vi "Angular PID Controller.vi"(8 "error in":errorcluster) -> ()   [LabVIEW 2015]
doc: "This VI executes continuously carrying out the current operation and responding to updates or new operations. It will often contain the timing or control code that is difficult to place directly in TeleOp. This VI generally opens all sensors and motors and isolates the rest of the robot code from knowing how the operations are carried out."
uses:
  <vilib>/Rock Robotics/WPI/CAN/TalonSRX/WPI_CANTalonSRX_GlobalStatus.ctl
  <vilib>/Rock Robotics/WPI/MotorControl/WPI_MotorControlOpenCANTalonSRX.vi
  Angular PID Setpoints.ctl
  Angular PID Operations.ctl
  <vilib>/Rock Robotics/WPI/CAN/TalonSRX/WPI_CANTalonSRX_APIControlMode.ctl
  <vilib>/Rock Robotics/WPI/CAN/TalonSRX/WPI_CANTalonSRX_APIFeedbackSelect.ctl
  <vilib>/Rock Robotics/Network Tables/NT Write Boolean.vi
panel:
  out "Out F":dbl
  out "Out I Zone":dbl
  out "Out Ramp Rate":dbl
  out "Out D":dbl
  out "Out I":dbl
  out "Out P":dbl
  in  "Ramp Rate":dbl format="%#_13g"
  in  "I Zone":dbl format="%#_13g"
  in  "F":dbl format="%#_13g"
  in  "D":dbl format="%#_13g"
  in  "I":dbl=0.03 format="%#_13g"
  in  "P":dbl=3.0 format="%#_13g"
  in  "Update PID":bool
  out "Talon SRX Status 2":T1
  out "Current Rev":dbl
  out "Talon SRX Status":T1
  out "Set OutPut":dbl
  out "Current\nCmd":string
  # "Tip: It may be helpful to observe inputs and sensor values.\nYou may also want to display tuning or debugging controls."
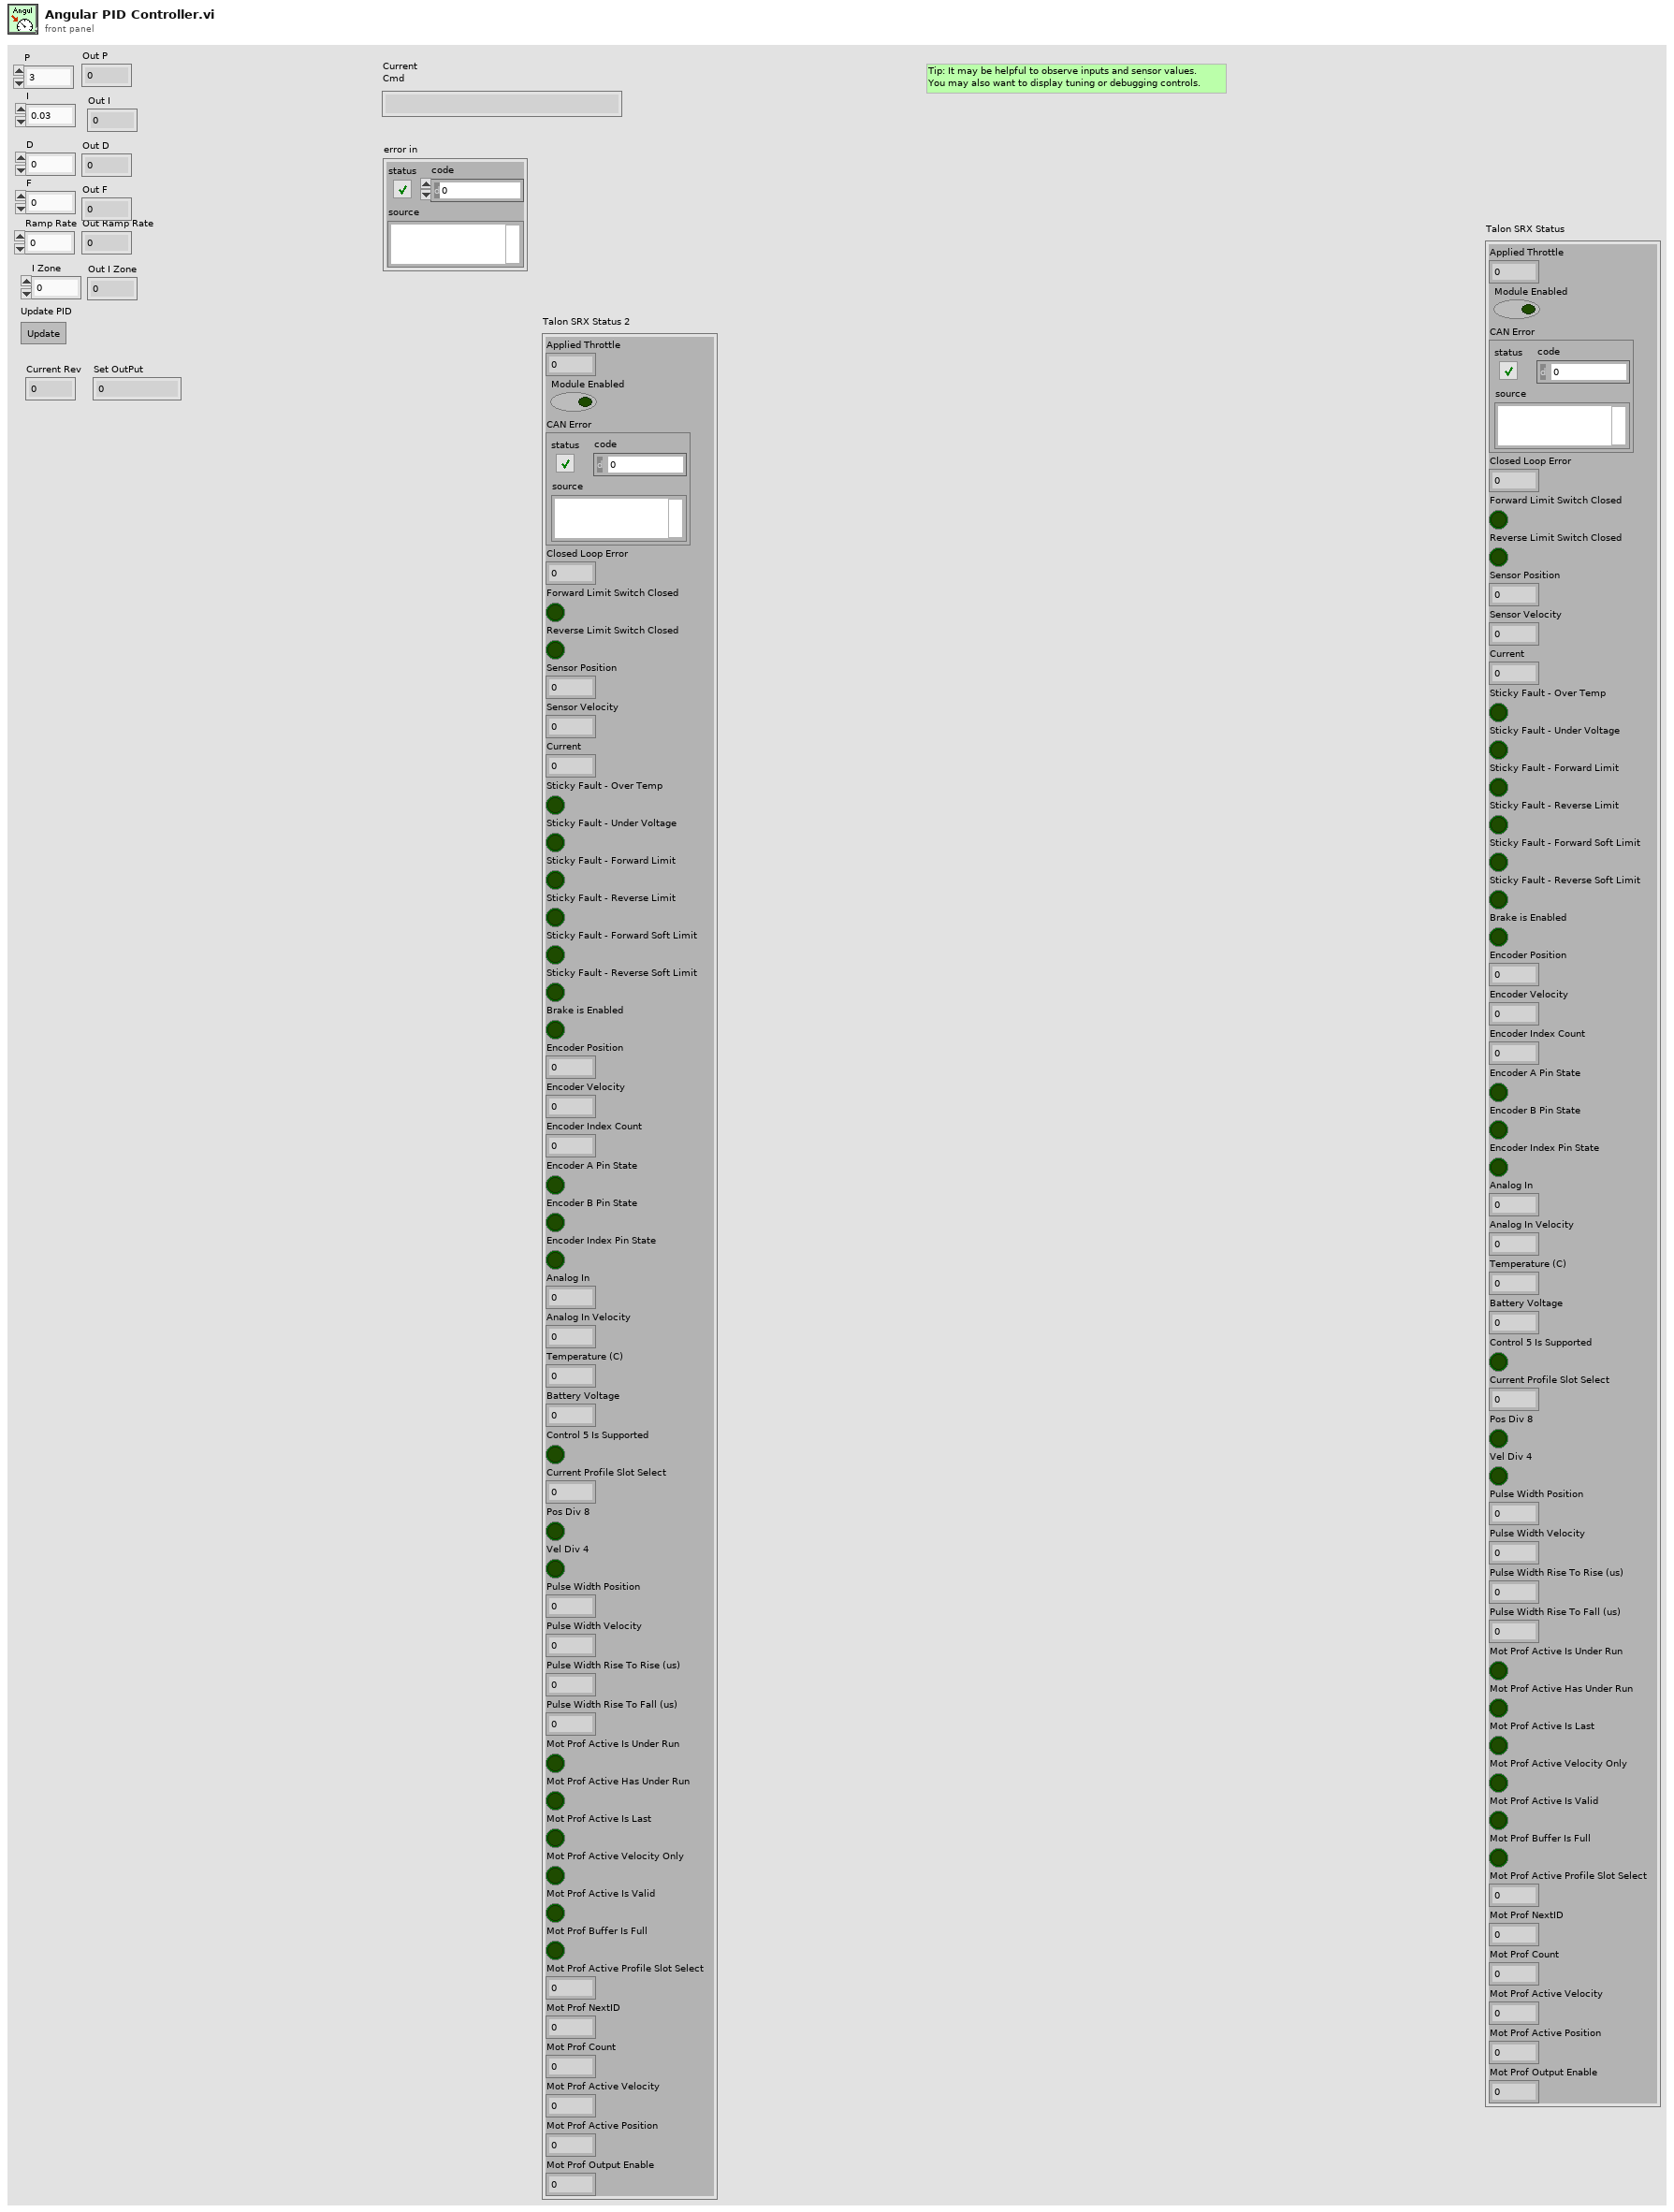
[diagram p1: front panel]
types:
  T1 = typedef "WPI_CANTalonSRX_GlobalStatus.ctl" = cluster{"Applied Throttle":dbl, "Module Enabled":bool, "CAN Error":errorcluster, "Closed Loop Error":dbl, "Forward Limit Switch Closed":bool, "Reverse Limit Switch Closed":bool, "Sensor Position":dbl, "Sensor Velocity":dbl, "Current":dbl, "Sticky Fault - Over Temp":bool, "Sticky Fault - Under Voltage":bool, "Sticky Fault - Forward Limit":bool, "Sticky Fault - Reverse Limit":bool, "Sticky Fault - Forward Soft Limit":bool, "Sticky Fault - Reverse Soft Limit":bool, "Brake is Enabled":bool, "Encoder Position":dbl, "Encoder Velocity":dbl, "Encoder Index Count":dbl, "Encoder A Pin State":bool, "Encoder B Pin State":bool, "Encoder Index Pin State":bool, "Analog In":dbl, "Analog In Velocity":dbl, "Temperature (C)":dbl, "Battery Voltage":dbl, "Control 5 Is Supported":bool, "Current Profile Slot Select":dbl, "Pos Div 8":bool, "Vel Div 4":bool, "Pulse Width Position":i32, "Pulse Width Velocity":i32, "Pulse Width Rise To Rise (us)":i32, "Pulse Width Rise To Fall (us)":i32, "Mot Prof Active Is Under Run":bool, "Mot Prof Active Has Under Run":bool, "Mot Prof Active Is Last":bool, "Mot Prof Active Velocity Only":bool, "Mot Prof Active Is Valid":bool, "Mot Prof Buffer Is Full":bool, "Mot Prof Active Profile Slot Select":i32, "Mot Prof NextID":i32, "Mot Prof Count":i32, "Mot Prof Active Velocity":dbl, "Mot Prof Active Position":dbl, "Mot Prof Output Enable":i32}
  T2 = typedef "WPI_CANTalonSRX_APIFeedbackSelect.ctl" = enum16{"Digital Quadrature Encoder", "Analog Potentiometer", "Analog Encoder", "Count on Quad-A (Rising-Edge)", "Count on Quad-A (Falling-Edge)", "CTR Magnetic Enc (Absolute)", "CTR Magnetic Enc (Relative)", "Pulse Width"}
  T3 = typedef "WPI_CANTalonSRX_APIControlMode.ctl" = enum8{"Percent VBus", "Speed", "Position", "Slave", "Unchanged / Invalid", "Voltage Compensation", "Current", "Motion Profile"}
  T4 = typedef "Angular PID Setpoints.ctl" = cluster{"Operation":T5, "Setpoint":dbl, "Duration":dbl}
  T5 = typedef "Angular PID Operations.ctl" = enum16{"Reserve", "Read Current", "Immediate", "Turn To Angle"}
  T6 = typedef "WPI_MotorControlDeviceRef.ctl" = cluster{"DeviceStatus":errorcluster, "Type":T7, "PWM":cluster{"PWM Channel":T8, "DeadBand":T9}, "CAN":cluster{"Device Number":u8, "Control Mode":T10, "Semaphore":T11, "Max Vout":dbl, "TalonSRX Control Mode":T3}, "Invert":bool}
  T7 = typedef "WPI_MotorControlType.ctl" = enum16{"PWM", "CAN", "CANTalonSRX"}
  T8 = typedef "FPGA_DIOPWMChannel.ctl" = enum8{"PWM 0", "PWM 1", "PWM 2", "PWM 3", "PWM 4", "PWM 5", "PWM 6", "PWM 7", "PWM 8", "PWM 9", "PWM MXP 0", "PWM MXP 1", "PWM MXP 2", "PWM MXP 3", "PWM MXP 4", "PWM MXP 5", "PWM MXP 6", "PWM MXP 7", "PWM MXP 8", "PWM MXP 9", "Invalid"}
  T9 = typedef "WPI_PWMDeadband.ctl" = cluster{"Name":string, "maxPositivePwm":i32, "minPositivePwm":i32, "centerPwm":i32, "maxNegativePwm":i32, "minNegativePwm":i32, "angularRange":u16}
  T10 = typedef "WPI_CANJaguar_ControlMode.ctl" = enum8{"Percent VBus", "Current", "Speed", "Position", "Voltage"}
  T11 = typedef "Semaphore RefNum" = refnum<k1>
  T12 = typedef "Command Status Info.ctl" = cluster{"Name":string, "Status":T13, "notifier out":T14}
  T13 = typedef "Completion Status.ctl" = enum16{"Successful", "Aborted", "Incomplete"}
  T14 = typedef "Completion Notifier.ctl" = refnum<notifier>
  T15 = cluster{"Default Command":T4, "Command Timing":cluster{"Start Time (ms)":u32, "Iterations":i32}, "Command Arguments":cluster{"Command Info":T12, "Description":string, "Default Command":T4, "notifier out":refnum<notifier>, "Subsystem Name":string}}
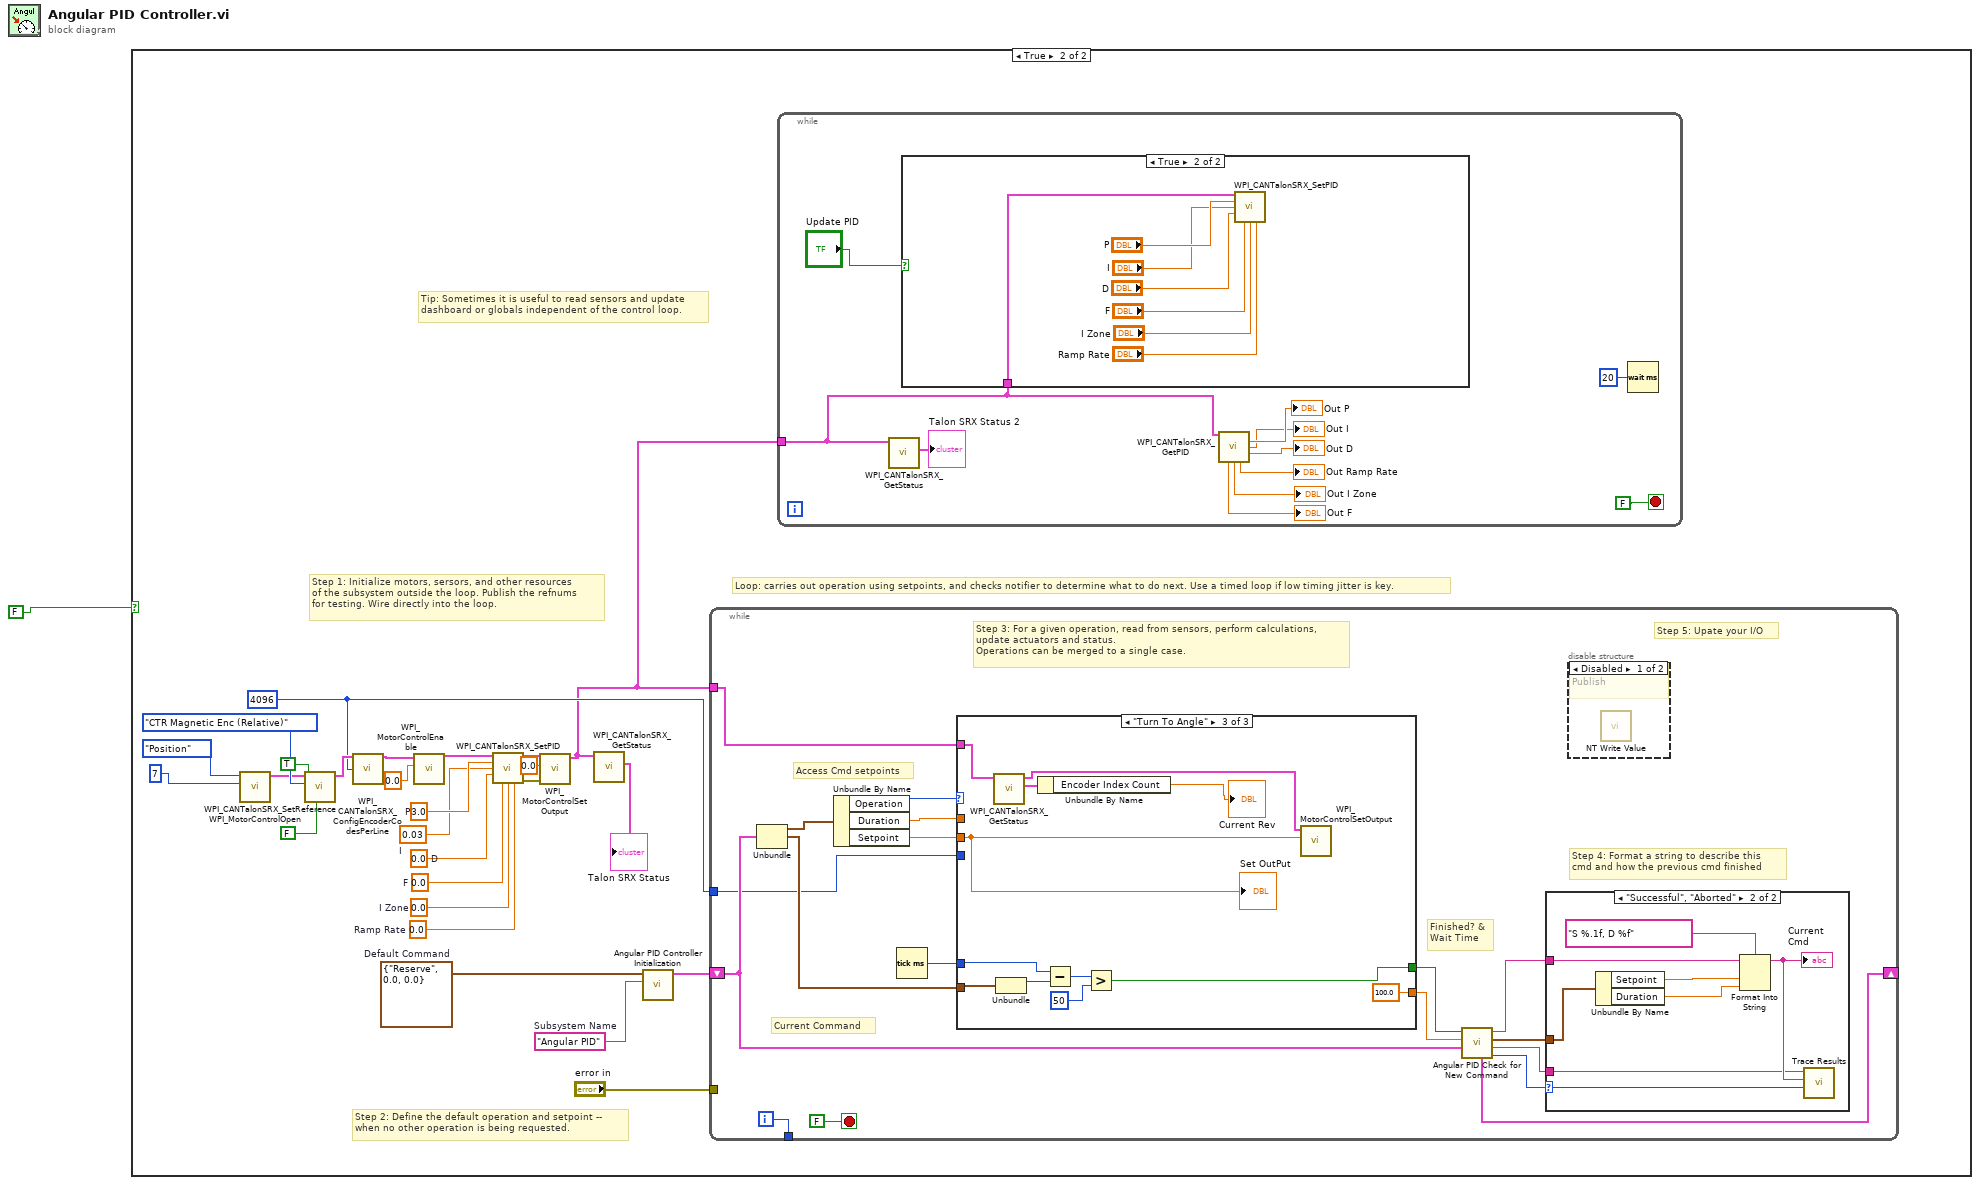
[diagram p0: block diagram]
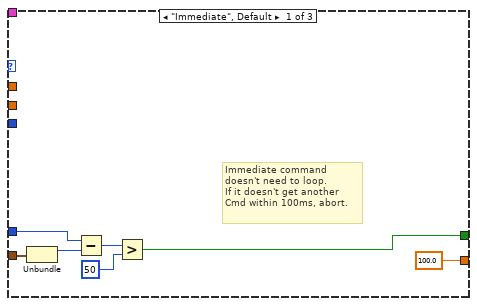
[diagram p6: hidden frame]
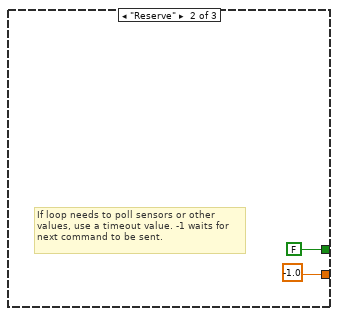
[diagram p7: hidden frame]
diagram:
  n1 = case shown="True" FALSE {
    frame False {
    }
    frame True {
      w10 = 0.0  # Ramp Rate
      w11 = 0.0  # I Zone
      w12 = 0.0  # F
      w13 = 0.0  # D
      w14 = 0.03  # I
      w15 = 3.0  # P
      w8 = u32 4096 ("Number Encoder Lines\n(Counts Per Rotation)")
      w24 = T4 {"Operation"=enum."Reserve", "Setpoint"=0.0, "Duration"=0.0}  # Default Command
      w25 = "Angular PID"  # Subsystem Name
      # "Tip: Sometimes it is useful to read sensors and update\ndashboard or globals independent of the control loop."
      # "Step 2: Define the default operation and setpoint --\nwhen no other operation is being requested."
      # "Step 1: Initialize motors, sersors, and other resources\nof the subsystem outside the loop. Publish the refnums\nfor testing. Wire directly into the loop."
      # "Loop: carries out operation using setpoints, and checks notifier to determine what to do next. Use a timed loop if low timing jitter is key."
      n2 = call-poly <vilib>:"WPI_MotorControlOpen.vi"("Device Number"=u8 7, "Control Mode"=WPI_CANTalonSRX_APIControlMode."Position") -> ("MotorControlDeviceRef"=w20:T6)  [unwired: 8 in, 1 out]
      n3 = call <vilib>:"WPI_CANTalonSRX_SetReference.vi"("Reverse Closed-Loop Output"=FALSE, "Reverse Feedback Sensor"=TRUE, "Feedback Reference"=WPI_CANTalonSRX_APIFeedbackSelect."CTR Magnetic Enc (Relative)", "CAN Talon SRX Ref"=w20) -> ("CAN Talon SRX Ref"=w19:T6)  [unwired: 6 in, 1 out]
      n4 = call <vilib>:"WPI_CANTalonSRX_ConfigEncoderCodesPerLine.vi"("CAN Talon SRX Ref"=w19, "Number Encoder Lines\n(Counts Per Rotation)"=w8) -> ("CAN Talon SRX Ref"=w18:T6)  [unwired: 12 in, 1 out]
      n5 = call <vilib>:"WPI_MotorControlEnable.vi"("Encoder Initial Position"=0.0, "CAN MotorDevRef"=w18) -> ("CAN MotorDevRef"=w16:T6)  [unwired: 8 in, 1 out]
      n6 = call <vilib>:"WPI_CANTalonSRX_SetPID.vi"("CAN Talon SRX Ref"=w16, "P"=w15, "I"=w14, "D"=w13, "F"=w12, "I Zone"=w11, "Ramp Rate"=w10) -> ("CAN Talon SRX Ref"=w6:T6, "error out"=w7:errorcluster)  [unwired: 7 in]
      n7 = call <vilib>:"WPI_MotorControlSetOutput.vi"("error in (no error)"=w7, "Output"=0.0, "MotorControlDevRef"=w6) -> ("MotorControlDevRef"=w3:T6)  [unwired: 6 in, 2 out]
      n8 = call <vilib>:"WPI_CANTalonSRX_GetStatus.vi"("CAN Talon SRX Ref"=w3) -> ("Talon SRX Status"=→"Talon SRX Status":T1)  [unwired: 8 in, 2 out]
      n9 = call "Angular PID Controller Initialization.vi"("Subsystem Name"=w25, "Default Command"=w24) -> ("Command Info"=w26:T15)  [unwired: 9 in]
      n10 = while {
        shift-right: [w54] -> _
        shift-left: w26 -> [w55]
        tunnel: [w62] -> _
        tunnel: "error in" -> [_]
        tunnel: w3 -> [w47]
        tunnel: w8 -> [w46]
        i -> [w62]
        stop <- FALSE stop-if-true
        # "Step 5: Upate your I/O"
        # "Step 4: Format a string to describe this\ncmd and how the previous cmd finished"
        # "Current Command"
        # "Access Cmd setpoints"
        # "Finished? &\nWait Time"
        # "Step 3: For a given operation, read from sensors, perform calculations,\nupdate actuators and status.\nOperations can be merged to a single case."
        n11 = Unbundle(w55) -> ("Default Command"=w61:T4, "Command Timing"=w57:cluster{"Start Time (ms)":u32, "Iterations":i32})  [unwired: 1 out]
        n12 = Unbundle By Name(w61) -> ("Operation"=w60:T5, "Duration"=w59:dbl, "Setpoint"=w56:dbl)
        n13 = Tick Count (ms)() -> (millisecond timer value=w58:u32)
        n14 = case shown="\"Turn To Angle\"" w60 {
          tunnel: [100.0 -1.0 100.0] -> w52
          tunnel: [w72 FALSE ("ignore previous (F)") w81] -> w53
          tunnel: w57 -> [w74 _ w82]
          tunnel: w59 -> [_ _ _]
          tunnel: w58 -> [w73 _ w83]
          tunnel: w56 -> [_ _ w89]
          tunnel: w47 -> [_ _ w91]
          tunnel: w46 -> [_ _ _]
          frame "Immediate", Default {
            # "Immediate command\ndoesn't need to loop.\nIf it doesn't get another\nCmd within 100ms, abort."
            n15 = Unbundle(w74) -> ("Start Time (ms)"=w77:u32)  [unwired: 1 out]
            n16 = Subtract(x=w73, y=w77) -> (x-y=w76:u32)
            n17 = Greater?(x=w76, y=u8 50 ("Left Motor")) -> (0:w72:bool)
          }
          frame "Reserve" {
            # "If loop needs to poll sensors or other\nvalues, use a timeout value. -1 waits for\nnext command to be sent."
          }
          frame "Turn To Angle" {
            n18 = call <vilib>:"WPI_CANTalonSRX_GetStatus.vi"("CAN Talon SRX Ref"=w91) -> ("Talon SRX Status"=w90:T1, "CAN Talon SRX Ref"=w88:T6)  [unwired: 8 in, 1 out]
            n19 = Unbundle(w82) -> ("Start Time (ms)"=w86:u32)  [unwired: 1 out]
            n20 = Unbundle By Name(w90) -> ("Encoder Index Count"=→"Current Rev":dbl)
            n21 = Subtract(x=w83, y=w86) -> (x-y=w85:u32)
            n22 = Greater?(x=w85, y=u8 50 ("Left Motor")) -> (0:w81:bool)
            n23 = call <vilib>:"WPI_MotorControlSetOutput.vi"("Output"=w89, "MotorControlDevRef"=w88) -> ()  [unwired: 7 in, 3 out]
            "Set OutPut" <- w89
          }
        }
        n24 = call "Angular PID Check for New Command.vi"("Current Command"=w55, "Wait time (ms)"=w52, "Finished?"=w53) -> ("Completion"=w48:T13, "Subsystem Name"=w49:string, "Current Command"=w50:T4, "Initial Trace String"=w51:string, "NextCommand"=w54:T15)  [unwired: 4 in]
        n25 = case shown="\"Successful\", \"Aborted\"" w48 {
          selector: w48 -> [_ w71]
          tunnel: w51 -> [_ w67]
          tunnel: w50 -> [_ w68]
          tunnel: w49 -> [_ w64]
          frame "Incomplete", Default {
            # "Continuing current command"
          }
          frame "Successful", "Aborted" {
            # "Report and setup for next command"
            n26 = Unbundle By Name(w68) -> ("Setpoint"=w70:dbl, "Duration"=w65:dbl)
            n27 = Format Into String(format string="S %.1f, D %f", initial string=w67, w70, w65) -> (resulting string=w66:string)  [unwired: 1 in, 1 out]
            "Current\nCmd" <- w66
            n28 = call <vilib>:"Trace Results.vi"("Status of previous command"=w71, "Description"=w66, "Subsystem"=w64) -> ()  [unwired: 9 in]
          }
        }
        n29 = disable-structure shown="Disabled" {
          frame Disabled {
            # "Publish"
            n30 = call-poly <vilib>:"NT Write Value.vi"() -> ()  [unwired: 11 in, 1 out]
          }
          frame Enabled {
          }
        }
      }
      n31 = while {
        tunnel: w3 -> [w34]
        stop <- FALSE stop-if-true
        n32 = call <vilib>:"WPI_CANTalonSRX_GetStatus.vi"("CAN Talon SRX Ref"=w34) -> ("Talon SRX Status"=→"Talon SRX Status 2":T1)  [unwired: 8 in, 2 out]
        n33 = case shown="True" "Update PID" {
          tunnel: w34 -> [_ w39]
          frame False {
          }
          frame True {
            n34 = call <vilib>:"WPI_CANTalonSRX_SetPID.vi"("CAN Talon SRX Ref"=w39, "P"="P", "I"="I", "D"="D", "F"="F", "I Zone"="I Zone", "Ramp Rate"="Ramp Rate") -> ()  [unwired: 7 in, 2 out]
          }
        }
        n35 = call <vilib>:"WPI_CANTalonSRX_GetPID.vi"("CAN Talon SRX Ref"=w34) -> ("P"=→"Out P":dbl, "I"=→"Out I":dbl, "D"=→"Out D":dbl, "F"=→"Out F":dbl, "I Zone"=→"Out I Zone":dbl, "Ramp Rate"=→"Out Ramp Rate":dbl)  [unwired: 7 in, 2 out]
        n36 = Wait (ms)(milliseconds to wait=u32 20) -> ()  [unwired: 1 out]
      }
    }
  }
